vi "Aim drawings.vi"(1 "Particle Scores":T2, 2 "Processed Image":T1(plugin-control), 3 "Calculated height [m]":dbl, 4 "Center target position real life height [m]":dbl, 5 "Center target position Y":dbl, 6 "Y ratio":dbl) -> (0 "Processed Image + aim markings":T1(plugin-control))   [LabVIEW 2012]
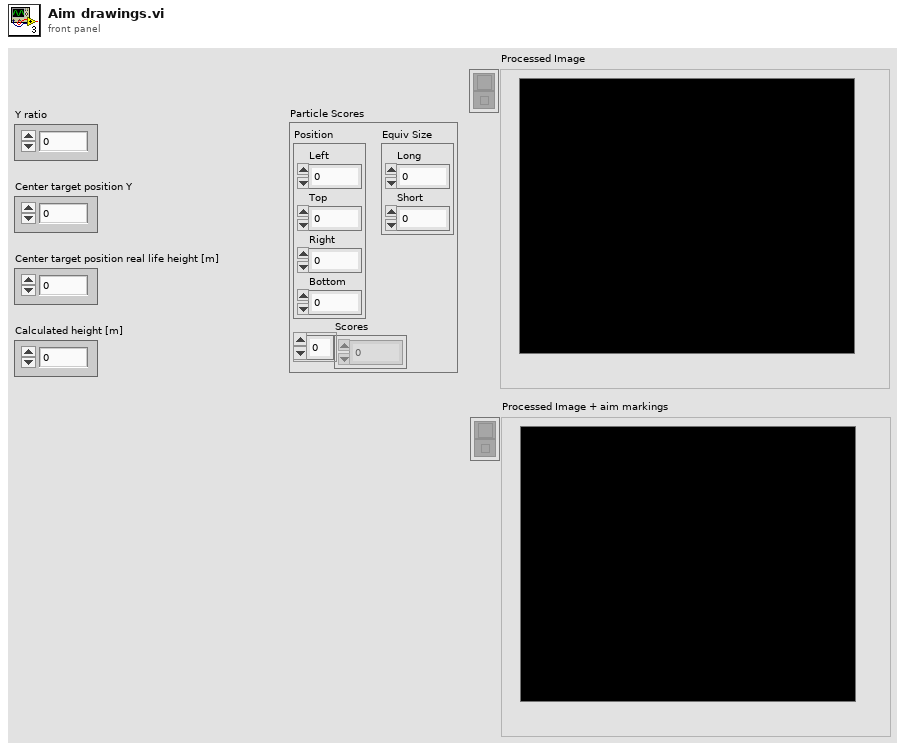
[diagram p1: front panel]
types:
  T1 = typedef "IMAQ Image.ctl" = refnum<image>
  T2 = cluster{"Position":cluster{"Left":dbl, "Top":dbl, "Right":dbl, "Bottom":dbl}, "Scores":dbl[], "Equiv Size":cluster{"Long":dbl, "Short":dbl}}
  T3 = cluster{"Left":dbl, "Top":dbl, "Right":dbl, "Bottom":dbl}
  T4 = cluster{"Left":i32, "Top":i32, "Right":i32, "Bottom":i32}
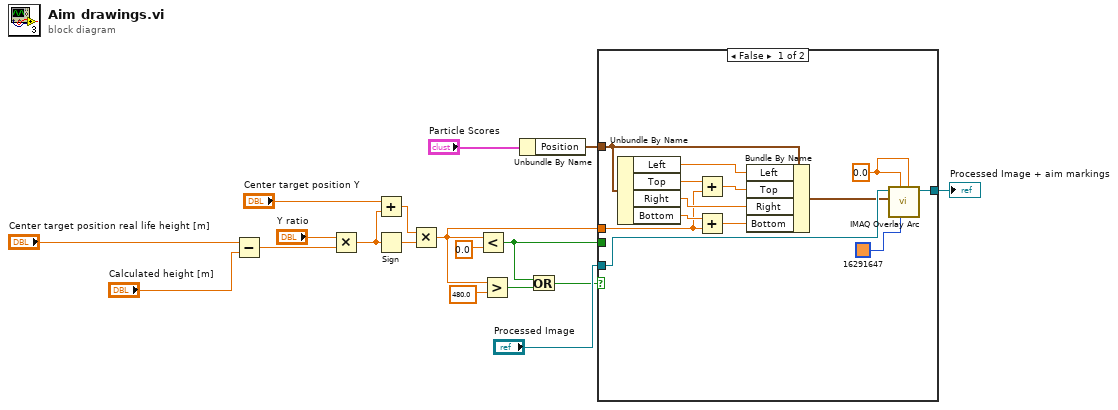
[diagram p0: block diagram]
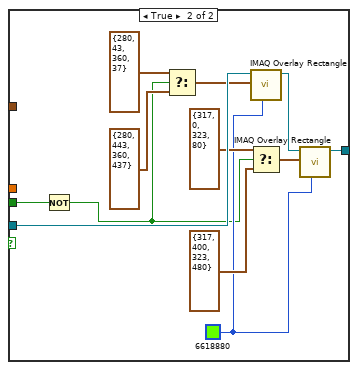
[diagram p2: hidden frame]
diagram:
  n1 = Subtract(x="Center target position real life height [m]", y="Calculated height [m]") -> (x-y=w6:dbl)
  n2 = Multiply(x="Y ratio", y=w6) -> (x*y=w4:dbl)
  n3 = Add(x="Center target position Y", y=w4) -> (x+y=w5:dbl)
  n4 = Sign(1:w4) -> (0:w3:dbl)
  n5 = Multiply(x=w5, y=w3) -> (x*y=w1:dbl)
  n6 = Less?(x=w1, y=0.0) -> (x < y?=w12:bool)
  n7 = Greater?(x=w1, y=480.0) -> (0:w14:bool)
  n8 = Unbundle By Name("Particle Scores") -> ("Position"=w11:T3)
  n9 = Or(x=w12, y=w14) -> (x .or. y?=w16:bool)
  n10 = case shown="False" w16 {
    tunnel: w12 -> [_ w40]
    tunnel: [w20 w42] -> w2
    tunnel: "Processed Image" -> [w30 w41]
    tunnel: w11 -> [w27 _]
    tunnel: w1 -> [w24 _]
    frame False {
      w31 = 0.0 ("End Angle (degrees)")
      n11 = Unbundle By Name(w27) -> ("Left"=w26:dbl, "Top"=w28:dbl, "Right"=w25:dbl, "Bottom"=w29:dbl)
      n12 = Add(x=w28, y=w24) -> (x+y=w22:dbl)
      n13 = Add(x=w29, y=w24) -> (x+y=w23:dbl)
      n14 = Bundle By Name(cluster=w27, "Left"=w26, "Top"=w22, "Right"=w25, "Bottom"=w23) -> (w21:T3)
      n15 = call "IMAQ Overlay Arc"("End Angle (degrees)"=w31, "Color"=u32 16291647, "Start Angle (degrees)"=w31, "Bounding Rectangle"=w21, "Image"=w30) -> ("Image Out"=w20:T1)  [unwired: 5 in, 1 out]
    }
    frame True {
      w33 = u32 6618880 ("Color")
      n16 = Not(x=w40) -> (.not. x?=w32:bool)
      n17 = Select(t=T4 {"Left"=280, "Top"=43, "Right"=360, "Bottom"=37} ("Rectangle"), s=w32, f=T4 {"Left"=280, "Top"=443, "Right"=360, "Bottom"=437} ("Rectangle")) -> (s? t:f=w35:T4)
      n18 = call "IMAQ Overlay Rectangle"("Color"=w33, "Rectangle"=w35, "Image"=w41) -> ("Image Out"=w43:T1)  [unwired: 7 in, 1 out]
      n19 = Select(t=T4 {"Left"=317, "Top"=0, "Right"=323, "Bottom"=80} ("Rectangle"), s=w32, f=T4 {"Left"=317, "Top"=400, "Right"=323, "Bottom"=480} ("Rectangle")) -> (s? t:f=w34:T4)
      n20 = call "IMAQ Overlay Rectangle"("Color"=w33, "Rectangle"=w34, "Image"=w43) -> ("Image Out"=w42:T1)  [unwired: 7 in, 1 out]
    }
  }
  "Processed Image + aim markings" <- w2
